vi "Write Display - High Limit.vi"(8 "error in (no error)":errorcluster, 10 "high limit":dbl format="%#_13g", 11 "NT Scalar (Numeric) in":refnum<class "NT Scalar (Numeric).lvclass">) -> (0 "error out":errorcluster, 3 "NT Scalar (Numeric) out":refnum<class "NT Scalar (Numeric).lvclass">)   [LabVIEW 2020, in "PV Access.lvlib" / "PV Data.lvlib" / "NT Scalar (Numeric).lvclass"]
uses:
  NT Scalar (Numeric).lvclass
  NT Scalar (Numeric).lvclass/NT Scalar (Numeric).ctl
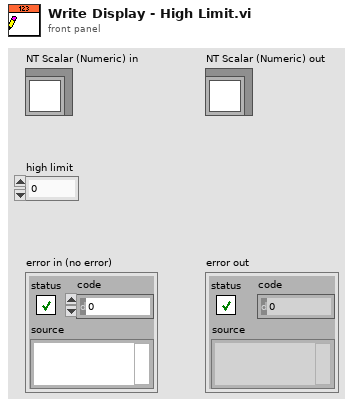
[diagram p1: front panel]
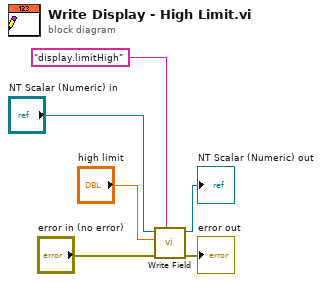
[diagram p0: block diagram]
diagram:
  n1 = call-dynamic "Write Field.vi"("field"="display.limitHigh", "error in (no error)"="error in (no error)", "value"="high limit", "Base Interface in"="NT Scalar (Numeric) in") -> ("error out"=→"error out":errorcluster, "Base Interface out"=→"NT Scalar (Numeric) out":refnum<class "NT Scalar (Numeric).lvclass">)  [unwired: 6 in]
